vi "CAN Talon Speed Control Encoder.vi"() -> ()   [LabVIEW 2015]
doc: "This example shows how to control motor speed using CAN Jaguar and a quadrature encoder. For details setting up and understanding CAN Jaguar, see the Can Jaguar Fundamentals tutorial accessable from the LabVIEW Getting Started Window.\n\nTo control the motor speed, a PID control loop runs on the Jaguar. Notice that the encoder is wired directly to the Jaguar. One advantage of this is that the PID control does not use resources on the roboRIO. One disadvantage is that the PID code cannot be viewed or changed. However, the control can be tuned by changing the PID Parameters.\n\nOn the diagram, notice that the PID tuning parameters are only applied once before the motor is enabled. To learn about changing PID parameters while the program is running, see the CAN Position Control Encoder example. Since the control loop runs on the Jaguar, the LabVIEW loop delay is set to a slow 100ms. In fact the only reason this loop needs to run is to send a new set speed and read the actual speed.\n\nCorrect tuning parameters for a PID controller are dependent on the complete system of the motor and the load. It will be difficult to tune this system if there is no load attached to the motor. While this example is not a PID tutorial, the following information may help in understanding how to tune your PID control system.\n\nP (proportional) depends on the present error, I (integral) on the accumulation of past errors, and D (derivative) is a prediction of future errors, based on the current rate of change. The proportional parameter (P) will reduce the rise time and will reduce, but never eliminate, the steady-state error. The integral parameter (I) will eliminate the steady-state error, but may make the transient response worse. The derivative parameter (D) will increase the stability of the system, reducing the overshoot, and improving the transient response. The effects of each parameter are summarized in a table on the front panel.\n\nThis example expects a USB cable connected from your development PC to the Type B USB Jack (next to the power input) on the roboRIO.\n\nThis example requires the Driver Station to be running with Teleoperated Enabled."
uses:
  <vilib>/Rock Robotics/WPI/CAN/TalonSRX/WPI_CANTalonSRX_APIControlMode.ctl
  <vilib>/Rock Robotics/WPI/CAN/TalonSRX/WPI_CANTalonSRX_APIFeedbackSelect.ctl
  <vilib>/Rock Robotics/WPI/MotorControl/WPI_MotorControlOpenCANTalonSRX.vi
panel:
  out "Thermometer 2":dbl(slide) scale=0.0..100.0
  out "Thermometer":dbl(slide) scale=0.0..100.0
  out "Speed of Wheel (RPM) 2":dbl(knob) scale=0.0..25000.0 scale format="%4d"
  out "Speed of Wheel (RPM)":dbl(knob) scale=0.0..25000.0 scale format="%4d"
  in  "Reverse Feedback Sensor 2":bool
  in  "I 2":dbl=0.001
  in  "F 2":dbl=2.5964
  in  "D 2":dbl
  in  "P 2":dbl=10.0
  out "Feedback Chart 3":cluster{dbl, dbl}(graph)
  out "Speed of Motor (RPM) 2":dbl(knob) scale=0.0..12000.0 scale format="%4d"
  in  "Set Speed (RPM) 2":dbl(slide) scale=-3000.0..3000.0
  in  "Reverse Feedback Sensor":bool
  out "Feedback Chart":cluster{dbl, dbl}(graph)
  in  "Device Number 2":u8=21
  in  "I":dbl=0.001
  in  "Encoder Codes Per Rev":u16=20
  in  "F":dbl=3.72
  in  "D":dbl
  in  "P":dbl=10.0
  in  "Set Speed (RPM)":dbl(slide) scale=0.0..12000.0
  out "Speed of Motor (RPM)":dbl(knob) scale=0.0..12000.0 scale format="%4d"
  in  "Device Number 1":u8=22
  in  "stop":bool
  # "Set these inputs before running."
  # "Tuning parameters"
  # "Feed-Forward"
  # "This can be set while running."
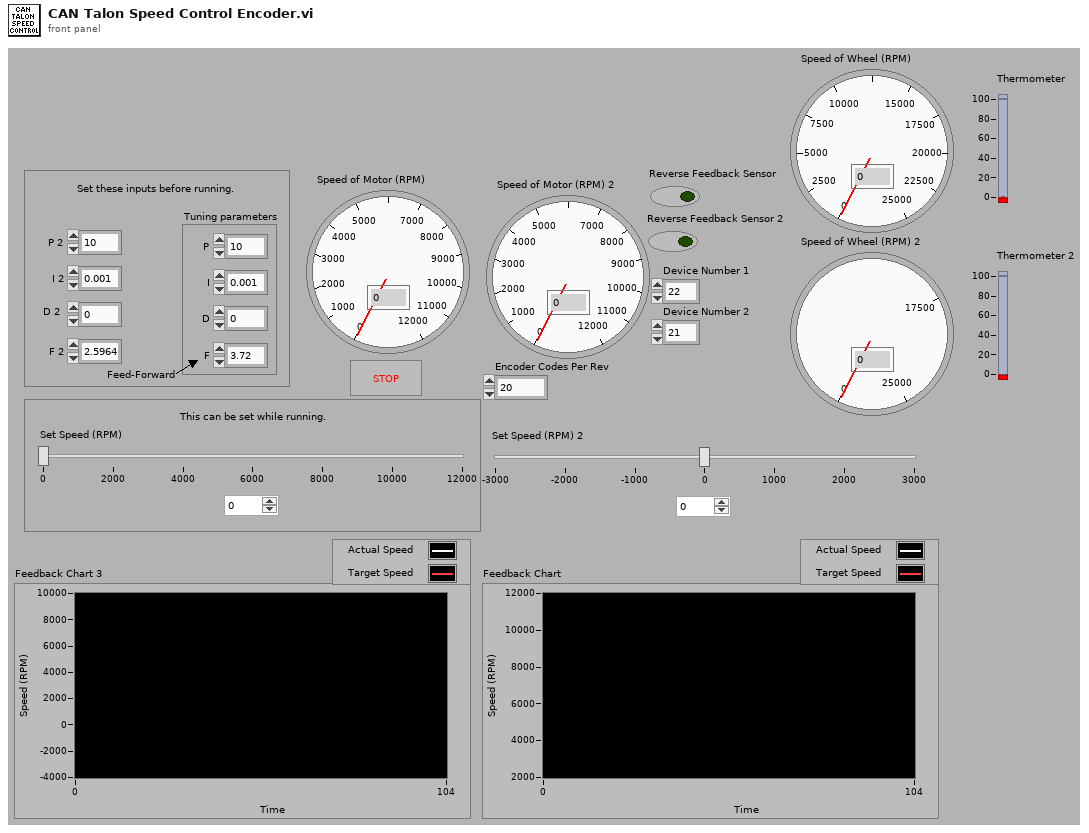
[diagram p1: front panel]
types:
  T1 = typedef "WPI_CANTalonSRX_APIFeedbackSelect.ctl" = enum16{"Digital Quadrature Encoder", "Analog Potentiometer", "Analog Encoder", "Count on Quad-A (Rising-Edge)", "Count on Quad-A (Falling-Edge)", "CTR Magnetic Enc (Absolute)", "CTR Magnetic Enc (Relative)", "Pulse Width"}
  T2 = typedef "WPI_CANTalonSRX_APIControlMode.ctl" = enum8{"Percent VBus", "Speed", "Position", "Slave", "Unchanged / Invalid", "Voltage Compensation", "Current", "Motion Profile"}
  T3 = typedef "WPI_MotorControlDeviceRef.ctl" = cluster{"DeviceStatus":errorcluster, "Type":T4, "PWM":cluster{"PWM Channel":T5, "DeadBand":T6}, "CAN":cluster{"Device Number":u8, "Control Mode":T7, "Semaphore":T8, "Max Vout":dbl, "TalonSRX Control Mode":T2}, "Invert":bool}
  T4 = typedef "WPI_MotorControlType.ctl" = enum16{"PWM", "CAN", "CANTalonSRX"}
  T5 = typedef "FPGA_DIOPWMChannel.ctl" = enum8{"PWM 0", "PWM 1", "PWM 2", "PWM 3", "PWM 4", "PWM 5", "PWM 6", "PWM 7", "PWM 8", "PWM 9", "PWM MXP 0", "PWM MXP 1", "PWM MXP 2", "PWM MXP 3", "PWM MXP 4", "PWM MXP 5", "PWM MXP 6", "PWM MXP 7", "PWM MXP 8", "PWM MXP 9", "Invalid"}
  T6 = typedef "WPI_PWMDeadband.ctl" = cluster{"Name":string, "maxPositivePwm":i32, "minPositivePwm":i32, "centerPwm":i32, "maxNegativePwm":i32, "minNegativePwm":i32, "angularRange":u16}
  T7 = typedef "WPI_CANJaguar_ControlMode.ctl" = enum8{"Percent VBus", "Current", "Speed", "Position", "Voltage"}
  T8 = typedef "Semaphore RefNum" = refnum<k1>
  T9 = typedef "WPI_CANTalonSRX_GlobalStatus.ctl" = cluster{"Applied Throttle":dbl, "Module Enabled":bool, "CAN Error":errorcluster, "Closed Loop Error":dbl, "Forward Limit Switch Closed":bool, "Reverse Limit Switch Closed":bool, "Sensor Position":dbl, "Sensor Velocity":dbl, "Current":dbl, "Sticky Fault - Over Temp":bool, "Sticky Fault - Under Voltage":bool, "Sticky Fault - Forward Limit":bool, "Sticky Fault - Reverse Limit":bool, "Sticky Fault - Forward Soft Limit":bool, "Sticky Fault - Reverse Soft Limit":bool, "Brake is Enabled":bool, "Encoder Position":dbl, "Encoder Velocity":dbl, "Encoder Index Count":dbl, "Encoder A Pin State":bool, "Encoder B Pin State":bool, "Encoder Index Pin State":bool, "Analog In":dbl, "Analog In Velocity":dbl, "Temperature (C)":dbl, "Battery Voltage":dbl, "Control 5 Is Supported":bool, "Current Profile Slot Select":dbl, "Pos Div 8":bool, "Vel Div 4":bool, "Pulse Width Position":i32, "Pulse Width Velocity":i32, "Pulse Width Rise To Rise (us)":i32, "Pulse Width Rise To Fall (us)":i32, "Mot Prof Active Is Under Run":bool, "Mot Prof Active Has Under Run":bool, "Mot Prof Active Is Last":bool, "Mot Prof Active Velocity Only":bool, "Mot Prof Active Is Valid":bool, "Mot Prof Buffer Is Full":bool, "Mot Prof Active Profile Slot Select":i32, "Mot Prof NextID":i32, "Mot Prof Count":i32, "Mot Prof Active Velocity":dbl, "Mot Prof Active Position":dbl, "Mot Prof Output Enable":i32}
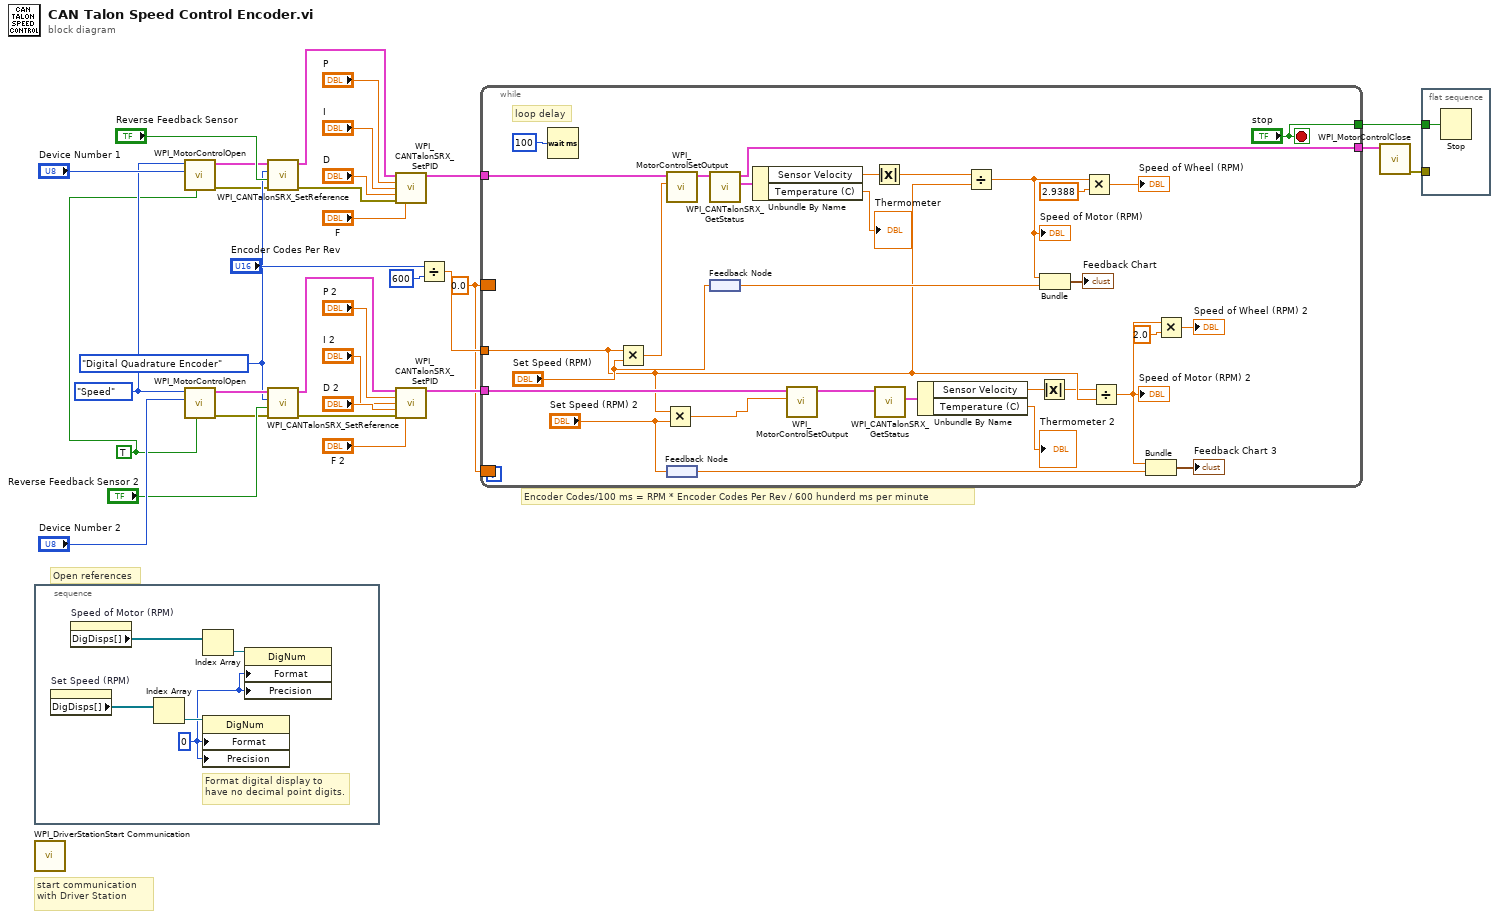
[diagram p0: block diagram]
diagram:
  w3 = TRUE ("Invert")
  w6 = WPI_CANTalonSRX_APIFeedbackSelect."Digital Quadrature Encoder" ("Feedback Reference")
  w5 = WPI_CANTalonSRX_APIControlMode."Speed" ("Control Mode")
  w4 = 0.0
  # "Open references"
  # "Encoder Codes/100 ms = RPM * Encoder Codes Per Rev / 600 hunderd ms per minute"
  # "start communication with Driver Station"
  n1 = stacked-sequence {
    frame #0 {
      w33 = u8 0 ("Display Format:Format")
      # "Format digital display to have no decimal point digits."
      n2 = property on="Set Speed (RPM)" class="Slide (strict)"() -> ("DigDisps[]"=w34:refnum<vi>[])  [unwired: 2 in, 2 out]
      n3 = property on="Speed of Motor (RPM)" class="Knob (strict)"() -> ("DigDisps[]"=w37:refnum<vi>[])  [unwired: 2 in, 2 out]
      n4 = Index Array(array=w34) -> (element=w35:refnum<vi>)  [unwired: 1 in]
      n5 = Index Array(array=w37) -> (element=w36:refnum<vi>)  [unwired: 1 in]
      n6 = property class="DigNum"(reference=w35, "Format"=w33, "Precision"=w33) -> ()  [unwired: 1 in, 2 out]
      n7 = property class="DigNum"(reference=w36, "Format"=w33, "Precision"=w33) -> ()  [unwired: 1 in, 2 out]
    }
  }
  n8 = call <vilib>:"WPI_DriverStationStart Communication.vi"() -> ()  [unwired: 2 in, 10 out]
  n9 = call-poly <vilib>:"WPI_MotorControlOpen.vi"("Invert"=w3, "Device Number"="Device Number 1", "Control Mode"=w5) -> ("error out"=w1:errorcluster, "MotorControlDeviceRef"=w2:T3)  [unwired: 2 in, 5 out]
  n10 = call-poly <vilib>:"WPI_MotorControlOpen.vi"("Invert"=w3, "Device Number"="Device Number 2", "Control Mode"=w5) -> ("error out"=w9:errorcluster, "MotorControlDeviceRef"=w8:T3)  [unwired: 2 in, 5 out]
  n11 = call <vilib>:"WPI_CANTalonSRX_SetReference.vi"("error in (no error)"=w1, "Reverse Feedback Sensor"="Reverse Feedback Sensor", "Feedback Reference"=w6, "CAN Talon SRX Ref"=w2) -> ("error out"=w18:errorcluster, "CAN Talon SRX Ref"=w21:T3)  [unwired: 6 in]
  n12 = call <vilib>:"WPI_CANTalonSRX_SetReference.vi"("error in (no error)"=w9, "Reverse Feedback Sensor"="Reverse Feedback Sensor 2", "Feedback Reference"=w6, "CAN Talon SRX Ref"=w8) -> ("error out"=w11:errorcluster, "CAN Talon SRX Ref"=w14:T3)  [unwired: 6 in]
  n13 = call <vilib>:"WPI_CANTalonSRX_SetPID.vi"("CAN Talon SRX Ref"=w21, "P"="P", "I"="I", "D"="D", "error in (no error)"=w18, "F"="F") -> ("CAN Talon SRX Ref"=w31:T3)  [unwired: 8 in, 1 out]
  n14 = call <vilib>:"WPI_CANTalonSRX_SetPID.vi"("CAN Talon SRX Ref"=w14, "P"="P 2", "I"="I 2", "D"="D 2", "error in (no error)"=w11, "F"="F 2") -> ("CAN Talon SRX Ref"=w7:T3)  [unwired: 8 in, 1 out]
  n15 = Divide(x="Encoder Codes Per Rev", y=u16 600) -> (x/y=w26:dbl)
  n16 = while {
    tunnel: ["stop"] -> w30
    tunnel: w31 -> [w65]
    tunnel: [w64] -> w32
    tunnel: w26 -> [w50]
    border: w4 -> [_]
    tunnel: w7 -> [w51]
    border: w4 -> [_]
    stop <- "stop" stop-if-true
    # "loop delay"
    n17 = Wait (ms)(milliseconds to wait=u32 100) -> ()  [unwired: 1 out]
    n18 = Multiply(x=w50, y="Set Speed (RPM)") -> (x*y=w39:dbl)
    n19 = Multiply(x=w50, y="Set Speed (RPM) 2") -> (x*y=w38:dbl)
    n20 = call <vilib>:"WPI_MotorControlSetOutput.vi"("Output"=w39, "MotorControlDevRef"=w65) -> ("MotorControlDevRef"=w63:T3)  [unwired: 7 in, 2 out]
    n21 = feedback #1() -> (w54:dbl)
    n22 = feedback-in #1("Set Speed (RPM) 2") -> ()
    n23 = call <vilib>:"WPI_CANTalonSRX_GetStatus.vi"("CAN Talon SRX Ref"=w63) -> ("Talon SRX Status"=w62:T9, "CAN Talon SRX Ref"=w64:T3)  [unwired: 8 in, 1 out]
    n24 = feedback #2() -> (w60:dbl)
    n25 = feedback-in #2("Set Speed (RPM)") -> ()
    n26 = Unbundle By Name(w62) -> ("Sensor Velocity"=w61:dbl, "Temperature (C)"=→"Thermometer":dbl)
    n27 = call <vilib>:"WPI_MotorControlSetOutput.vi"("Output"=w38, "MotorControlDevRef"=w51) -> ("MotorControlDevRef"=w57:T3)  [unwired: 7 in, 2 out]
    n28 = Absolute Value(x=w61) -> (abs(x)=w43:dbl)
    n29 = call <vilib>:"WPI_CANTalonSRX_GetStatus.vi"("CAN Talon SRX Ref"=w57) -> ("Talon SRX Status"=w56:T9)  [unwired: 8 in, 2 out]
    n30 = Unbundle By Name(w56) -> ("Sensor Velocity"=w55:dbl, "Temperature (C)"=→"Thermometer 2":dbl)
    n31 = Divide(x=w43, y=w50) -> (x/y=w45:dbl)
    "Speed of Motor (RPM)" <- w45
    n32 = Absolute Value(x=w55) -> (abs(x)=w42:dbl)
    n33 = Bundle(w45, w60) -> (→"Feedback Chart":cluster{dbl, dbl})  [unwired: 1 in]
    n34 = Multiply(x=w45, y=2.9388) -> (x*y=→"Speed of Wheel (RPM)":dbl)
    n35 = Divide(x=w42, y=w50) -> (x/y=w49:dbl)
    "Speed of Motor (RPM) 2" <- w49
    n36 = Bundle(w49, w54) -> (→"Feedback Chart 3":cluster{dbl, dbl})  [unwired: 1 in]
    n37 = Multiply(x=w49, y=2.0) -> (x*y=→"Speed of Wheel (RPM) 2":dbl)
  }
  n38 = call <vilib>:"WPI_MotorControlClose.vi"("MotorControlDevRef"=w32) -> ("error out"=w29:errorcluster)  [unwired: 10 in]
  n39 = flat-sequence {
    tunnel: w30 -> [w68]
    tunnel: w29 -> [_]
    frame #0 {
      n40 = Stop(stop? (T)=w68) -> ()
    }
  }
